vi "Button Toggle.vi"(11 "Button Input":bool) -> (3 "Toggled Output":bool)   [LabVIEW 2018]
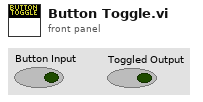
[diagram p1: front panel]
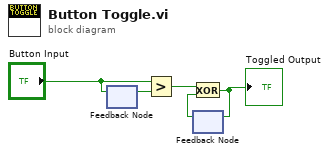
[diagram p0: block diagram]
diagram:
  n1 = feedback #1() -> (w3:bool)  [unwired: 1 in]
  n2 = feedback-in #1("Button Input") -> ()
  n3 = Greater?(x="Button Input", y=w3) -> (0:w2:bool)
  n4 = feedback #2() -> (w1:bool)  [unwired: 1 in]
  n5 = Exclusive Or(1:w1, 2:w2) -> (0:w4:bool)
  "Toggled Output" <- w4
  n6 = feedback-in #2(w4) -> ()
